vi "get modules in engine.vi"(8 "error in":errorcluster, 11 "engine mapping":refnum<data-value>) -> (0 "error out":errorcluster, 3 "Modules Configurations":refnum<class "TBM module configuration.lvclass">[](array[class]))   [LabVIEW 2013, in "PL Framework Configuration Tool.lvlib" / "Engine Mappings.lvclass"]
uses:
  Engine Mappings.lvclass
  <vilib>/NI/Tag Bus Module Framework/module configuration/TBM module configuration.lvclass
  Engine Parent/Read Modules Configurations.vi
  Engine Parent/Engine Parent Editor Node.lvclass
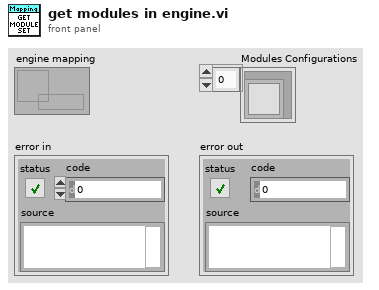
[diagram p1: front panel]
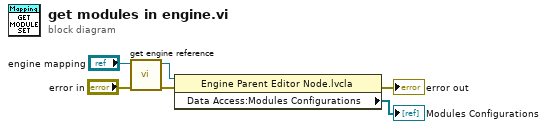
[diagram p0: block diagram]
diagram:
  n1 = call "get engine reference.vi"("error in"="error in", "engine mappings"="engine mapping") -> ("error out"=w4:errorcluster, "engine reference"=w3:refnum<data-value>)  [unwired: 8 in]
  n2 = property class="Engine Parent Editor Node.lvcla"(reference=w3, error in=w4) -> (error out=→"error out":errorcluster, "Data Access:Modules Configurations"=→"Modules Configurations":refnum<class "TBM module configuration.lvclass">[])  [unwired: 1 out]
